vi "io_bin_data_PCfile_to_instrument.vi"(7 "Source File":path, 8 "error in":errorcluster, 10 "Command (none)":string, 11 "VISA resource name":refnum<visa-resource-name>) -> (0 "error out":errorcluster, 3 "VISA resource name out":refnum<visa-resource-name>)   [LabVIEW 2014, in "rszvl_rsidr_core.lvlib"]
uses:
  rszvl_rsidr_core.lvlib
  type_Error_Codes.ctl
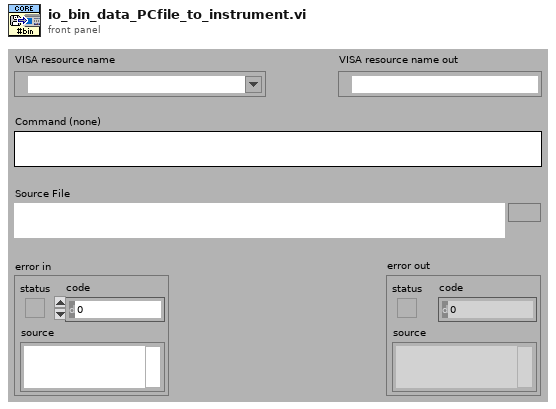
[diagram p1: front panel]
types:
  T1 = enum16{"open", "replace", "create", "open or create", "replace or create", "replace or create with confirmation"}
  T2 = typedef "rszvl_rsidr_core.lvlib/type_Error_Codes.ctl" = enum16{"No_error", "VISA_err_ResourceNotFound", "VISA_err_Timeout", "VISA_warn_MoreDataAvailable", "RS_err_MissingCallback", "RS_err_InvalidAttribute", "RS_err_InvalidValue", "RS_err_UnknownResource", "RS_err_AlreadyInitialized", "RS_err_InstrumentStatus", "RS_err_BadRepCapName", "RS_err_TypesMismatch", "RS_err_ValueNotSupported", "RS_err_InvalidRngTable", "RS_err_IDqueryFail", "RS_err_UnexpResponse", "VISA_warn_ConfigNotLoaded", "RS_err_AttributeNotReadable", "RS_err_AttributeNotWritable", "RS_err_InstrumentType", "RS_err_InstrumentOption", "VISA_err_InvalidSize", "RS_err_ReliabilityIndicator", "VISA_warn_UnknownStatus", "VISA_warn_TermCharRead", "VISA_err_IO_error"}
  T3 = typedef "rszvl_rsidr_core.lvlib/type_Session_Data.ctl" = cluster{"Instr type":string, "Instr type for err. msg.":string, "Installed Options":string[], "OPC Timeout":i32, "Query Instrument Status":bool, "Check Range":bool, "Check Options":bool, "Add LF to Write":bool, "Simulate":bool, "Logging":bool, "Logging params":variant, "Interface Type":enum16{"Unknown", "GPIB", "VXI", "GPIB_VXI", "ASRL", "PXI", "TCPIP", "USB", "SOCKET"}, "Fast Sweep":i32, "AdditionalFlags":i32, "WaitBeforeWrite":i32, "WaitBeforeRead":i32, "BinDataChunkSize":i64}
  T4 = enum16{"Unknown", "GPIB", "VXI", "GPIB_VXI", "ASRL", "PXI", "TCPIP", "USB", "SOCKET"}
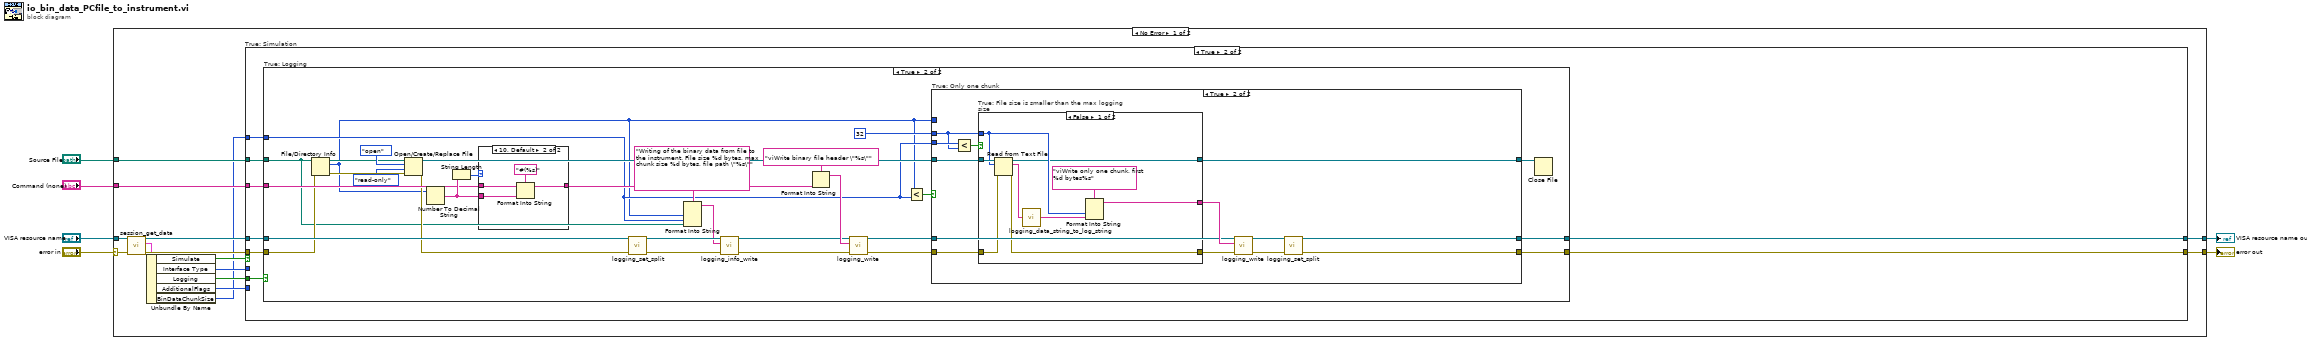
[diagram p0: block diagram]
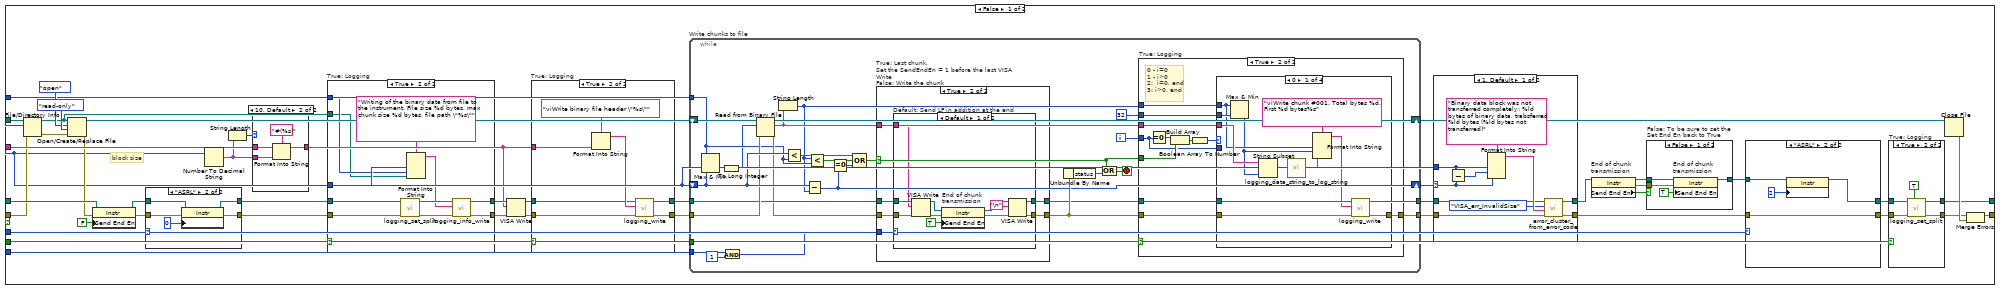
[diagram p2: hidden frame]
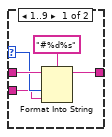
[diagram p7: hidden frame]
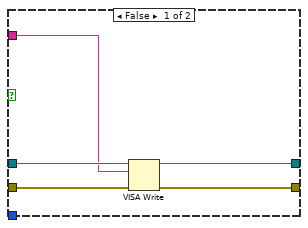
[diagram p9: hidden frame]
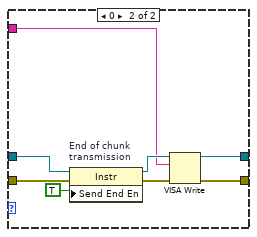
[diagram p10: hidden frame]
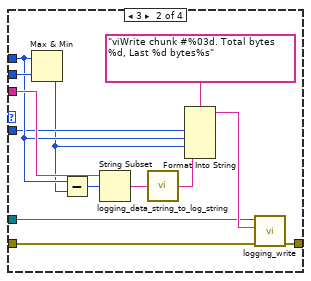
[diagram p12: hidden frame]
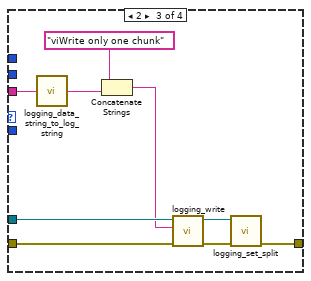
[diagram p13: hidden frame]
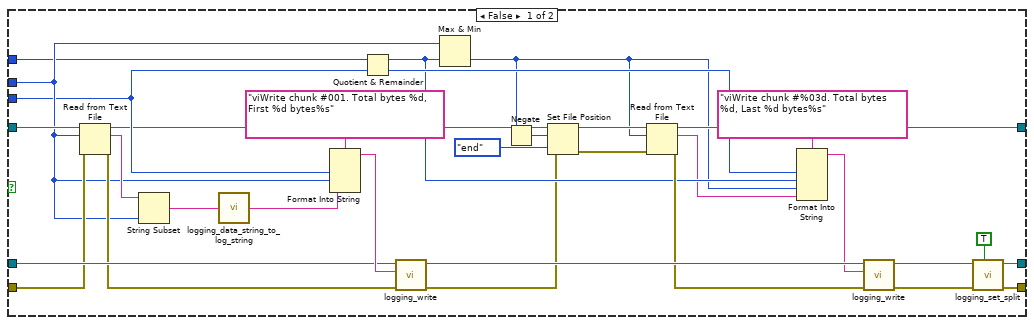
[diagram p18: hidden frame]
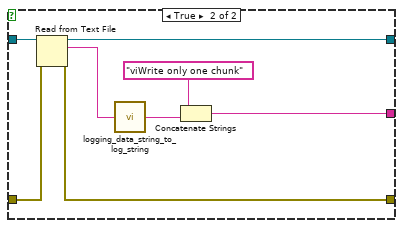
[diagram p19: hidden frame]
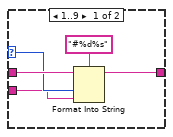
[diagram p20: hidden frame]
diagram:
  n1 = case shown="No Error" "error in" {
    selector: "error in" -> [w18 w348]
    tunnel: "Source File" -> [w20 _]
    tunnel: "Command (none)" -> [w19 _]
    tunnel: "VISA resource name" -> [w17 w349]
    tunnel: [w12 w348] -> w3
    tunnel: [w11 w349] -> w2
    frame No Error {
      n2 = call "session_get_data.vi"("error in"=w18, "VISA resource name"=w17) -> ("error out"=w16:errorcluster, "Session User Data out"=w14:T3, "VISA resource name out"=w15:refnum<visa-resource-name>)  [unwired: 7 in]
      n3 = Unbundle By Name(w14) -> ("Simulate"=w10:bool, "Interface Type"=w9:T4, "Logging"=w13:bool, "AdditionalFlags"=w8:i32, "BinDataChunkSize"=w7:i64)
      n4 = case "True: Simulation" shown="True" w10 {
        tunnel: w16 -> [w49 w241]
        tunnel: w15 -> [w65 w240]
        tunnel: w20 -> [w56 w239]
        tunnel: w19 -> [w52 w238]
        tunnel: [w29 w242] -> w11
        tunnel: [w30 w243] -> w12
        tunnel: w13 -> [w34 w244]
        tunnel: w7 -> [w35 w237]
        tunnel: w9 -> [w22 _]
        tunnel: w8 -> [w21 _]
        frame False {
          # "block size"
          n5 = File/Directory Info(path=w56, error in=w49) -> (path out=w44:path, size=w45:i64, error out=w53:errorcluster)  [unwired: 4 out]
          n6 = Open/Create/Replace File(file path (use dialog)=w44, error in=w53, operation (0:open)=T1."open", access (0:read/write)=enum16{"read/write", "read-only", "write-only"}."read-only") -> (refnum out=w62:refnum<file>, error out=w48:errorcluster)  [unwired: 2 in, 1 out]
          n7 = property on="Property Node" class="Instr"(reference=w65, error in=w48, "Send End En"=FALSE ("Message Based Settings:Send End Enable")) -> (reference out=w54:refnum<visa-resource-name>, error out=w55:errorcluster)
          n8 = case "4: ASRL" shown="\"ASRL\"" w22 {
            tunnel: w55 -> [w230 w235]
            tunnel: w54 -> [w231 w234]
            tunnel: [w231 w233] -> w47
            tunnel: [w230 w232] -> w46
            frame Default {
            }
            frame "ASRL" {
              n9 = property on="Property Node" class="Instr"(reference=w234, error in=w235, "Serial Settings:End Mode for Reads"=u16 0 ("ASRL End In")) -> (reference out=w233:refnum<visa-resource-name>, error out=w232:errorcluster)
            }
          }
          n10 = Number To Decimal String(number=w45) -> (decimal integer string=w51:string)  [unwired: 1 in]
          n11 = String Length(string=w51) -> (length=w50:i32)
          n12 = case shown="10, Default" w50 {
            selector: w50 -> [w102 _]
            tunnel: w52 -> [w103 w107]
            tunnel: w51 -> [w101 w105]
            tunnel: [w100 w106] -> w37
            frame 1..9 {
              n13 = Format Into String(format string="#%d%s", initial string=w103, w102, w101) -> (resulting string=w100:string)  [unwired: 1 in, 1 out]
            }
            frame 10, Default {
              n14 = Format Into String(format string="#(%s)", initial string=w107, w105) -> (resulting string=w106:string)  [unwired: 1 in, 1 out]
            }
          }
          n15 = case "True: Logging" shown="True" w34 {
            tunnel: w46 -> [w88 w99]
            tunnel: w47 -> [w87 w98]
            tunnel: w35 -> [_ w95]
            tunnel: [w88 w91] -> w41
            tunnel: [w87 w90] -> w42
            tunnel: w45 -> [_ w96]
            tunnel: w44 -> [_ w94]
            frame False {
            }
            frame True {
              n16 = call "logging_set_split.vi"("error in"=w99, "VISA resource name"=w98) -> ("error out"=w93:errorcluster, "VISA resource name out"=w92:refnum<visa-resource-name>)  [unwired: 8 in]
              n17 = Format Into String(format string="Writing of the binary data from file to the instrument. File size %d bytes, max chunk size %d bytes, file path \"%s\"", w96, w95, w94) -> (resulting string=w89:string)  [unwired: 2 in, 1 out]
              n18 = call "logging_info_write.vi"("error in"=w93, "String to write"=w89, "VISA resource name"=w92) -> ("error out"=w91:errorcluster, "VISA resource name out"=w90:refnum<visa-resource-name>)  [unwired: 7 in]
            }
          }
          n19 = VISA Write(VISA resource name=w42, write buffer=w37, error in (no error)=w41) -> (VISA resource name out=w39:refnum<visa-resource-name>, error out=w40:errorcluster)  [unwired: 1 out]
          n20 = case "True: Logging" shown="True" w34 {
            tunnel: w40 -> [w79 w84]
            tunnel: w39 -> [w78 w83]
            tunnel: [w79 w82] -> w38
            tunnel: [w78 w81] -> w36
            tunnel: w37 -> [_ w80]
            frame False {
            }
            frame True {
              n21 = Format Into String(format string="viWrite binary file header \"%s\"", w80) -> (resulting string=w85:string)  [unwired: 2 in, 1 out]
              n22 = call "logging_write.vi"("error in"=w84, "String to write"=w85, "VISA resource name"=w83) -> ("error out"=w82:errorcluster, "VISA resource name out"=w81:refnum<visa-resource-name>)  [unwired: 7 in]
            }
          }
          n23 = while "Write chunks to file" {
            tunnel: w38 -> [w142]
            tunnel: w36 -> [w134]
            tunnel: w35 -> [w125]
            shift-right: [w123] -> w59
            shift-left: w45 -> [w145]
            tunnel: [w140] -> w58
            shift-right: [w143] -> w61
            shift-left: w62 -> [w144]
            tunnel: w34 -> [w138]
            tunnel: [w130] -> w28
            tunnel: w21 -> [w127]
            i -> [w135]
            stop <- w146 stop-if-true
            n24 = Max & Min(x=w125, y=w145) -> (min(x,y)=w141:i64)  [unwired: 1 out]
            n25 = To Long Integer(number=w141) -> (32bit integer=w124:i32)
            n26 = And(x=w127, y=1 ("x")) -> (x .and. y?=w126:i32)
            n27 = Read from Binary File(8:w142, 10:w124, 11:w144) -> (0:w133:errorcluster, 2:w131:string, 3:w143:refnum<file>)  [unwired: 3 in, 1 out]
            n28 = String Length(string=w131) -> (length=w121:i32)
            n29 = Less?(x=w145, y=w125) -> (x < y?=w137:bool)
            n30 = Subtract(x=w145, y=w121) -> (x-y=w123:i64)
            n31 = Less?(x=w121, y=w125) -> (x < y?=w136:bool)
            n32 = Equal To 0?(x=w123) -> (x = 0?=w122:bool)
            n33 = Compound Arithmetic op=OR(w137, w136, w122) -> (w129:bool)
            n34 = case "True: Last chunk,\nSet the SendEndEn = 1 before the last VISA Write\nFalse: Write the chunk" shown="True" w129 {
              tunnel: w134 -> [w151 w158]
              tunnel: w133 -> [w152 w157]
              tunnel: [w150 w156] -> w132
              tunnel: w131 -> [w148 w155]
              tunnel: [w149 w154] -> w130
              tunnel: w126 -> [_ w153]
              frame False {
                n35 = VISA Write(VISA resource name=w151, write buffer=w148, error in (no error)=w152) -> (VISA resource name out=w149:refnum<visa-resource-name>, error out=w150:errorcluster)  [unwired: 1 out]
              }
              frame True {
                n36 = case "Default: Send LF in addition at the end" shown="Default" w153 {
                  tunnel: w158 -> [w163 w177]
                  tunnel: w157 -> [w164 w176]
                  tunnel: [w167 w173] -> w156
                  tunnel: w155 -> [w160 w172]
                  tunnel: [w166 w171] -> w154
                  frame Default {
                    n37 = VISA Write(VISA resource name=w163, write buffer=w160, error in (no error)=w164) -> (VISA resource name out=w161:refnum<visa-resource-name>, error out=w162:errorcluster)  [unwired: 1 out]
                    n38 = property on="End of chunk\ntransmission" class="Instr"(reference=w161, error in=w162, "Send End En"=TRUE ("Message Based Settings:Send End Enable")) -> (reference out=w168:refnum<visa-resource-name>, error out=w169:errorcluster)
                    n39 = VISA Write(VISA resource name=w168, write buffer="\n" ("Line Feed Constant"), error in (no error)=w169) -> (VISA resource name out=w166:refnum<visa-resource-name>, error out=w167:errorcluster)  [unwired: 1 out]
                  }
                  frame 0 {
                    n40 = property on="End of chunk\ntransmission" class="Instr"(reference=w177, error in=w176, "Send End En"=TRUE ("Message Based Settings:Send End Enable")) -> (reference out=w174:refnum<visa-resource-name>, error out=w175:errorcluster)
                    n41 = VISA Write(VISA resource name=w174, write buffer=w172, error in (no error)=w175) -> (VISA resource name out=w171:refnum<visa-resource-name>, error out=w173:errorcluster)  [unwired: 1 out]
                  }
                }
              }
            }
            n42 = Unbundle By Name(w132) -> ("status"=w147:bool)
            n43 = Compound Arithmetic op=OR(w129, w147) -> (w146:bool)
            n44 = case "True: Logging" shown="True" w138 {
              tunnel: w132 -> [w178 w189]
              tunnel: w130 -> [_ w188]
              tunnel: [w178 w187] -> w140
              tunnel: w131 -> [_ w186]
              tunnel: w121 -> [_ w185]
              tunnel: 32 ("length (rest)") -> [_ w184]
              tunnel: w129 -> [_ w183]
              tunnel: w135 -> [_ w179]
              frame False {
              }
              frame True {
                # "0 - i=0\n1 - i>0\n2:  i=0, end\n3: i>0, end"
                n45 = Equal To 0?(x=w179) -> (x = 0?=w182:bool)
                n46 = Build Array(w182, w183) -> (w181:bool[])
                n47 = Boolean Array To Number(Boolean array=w181) -> (number=w180:u32)
                n48 = case shown="0" w180 {
                  tunnel: w189 -> [w198 w211 w222 w223]
                  tunnel: w188 -> [w197 w210 w221 _]
                  tunnel: [w196 w201 w214 w223] -> w187
                  tunnel: w186 -> [w195 w209 w220 _]
                  tunnel: w185 -> [w192 w206 _ _]
                  tunnel: w184 -> [w193 w207 _ _]
                  tunnel: w179 -> [_ w204 _ _]
                  frame 0 {
                    n49 = Max & Min(x=w192, y=w193) -> (min(x,y)=w191:i32)  [unwired: 1 out]
                    n50 = String Subset(string=w195, length (rest)=w191) -> (substring=w194:string)  [unwired: 1 in]
                    n51 = call "logging_data_string_to_log_string.vi"("Raw string to log"=w194) -> ("Result log string"=w190:string)  [unwired: 4 in]
                    n52 = Format Into String(format string="viWrite chunk #001. Total bytes %d, First %d bytes%s", w192, w191, w190) -> (resulting string=w199:string)  [unwired: 2 in, 1 out]
                    n53 = call "logging_write.vi"("error in"=w198, "String to write"=w199, "VISA resource name"=w197) -> ("error out"=w196:errorcluster)  [unwired: 7 in, 1 out]
                  }
                  frame 3 {
                    n54 = Max & Min(x=w206, y=w207) -> (min(x,y)=w203:i32)  [unwired: 1 out]
                    n55 = Subtract(x=w206, y=w203) -> (x-y=w205:i32)
                    n56 = String Subset(string=w209, offset (0)=w205) -> (substring=w208:string)  [unwired: 1 in]
                    n57 = call "logging_data_string_to_log_string.vi"("Raw string to log"=w208) -> ("Result log string"=w202:string)  [unwired: 4 in]
                    n58 = Format Into String(format string="viWrite chunk #%03d. Total bytes %d, Last %d bytes%s", w204, w206, w203, w202) -> (resulting string=w212:string)  [unwired: 2 in, 1 out]
                    n59 = call "logging_write.vi"("error in"=w211, "String to write"=w212, "VISA resource name"=w210) -> ("error out"=w201:errorcluster)  [unwired: 7 in, 1 out]
                  }
                  frame 2 {
                    n60 = call "logging_data_string_to_log_string.vi"("Raw string to log"=w220) -> ("Result log string"=w217:string)  [unwired: 4 in]
                    n61 = Concatenate Strings("viWrite only one chunk" ("format string"), w217) -> (w218:string)
                    n62 = call "logging_write.vi"("error in"=w222, "String to write"=w218, "VISA resource name"=w221) -> ("error out"=w216:errorcluster, "VISA resource name out"=w215:refnum<visa-resource-name>)  [unwired: 7 in]
                    n63 = call "logging_set_split.vi"("error in"=w216, "VISA resource name"=w215) -> ("error out"=w214:errorcluster)  [unwired: 8 in, 1 out]
                  }
                  frame Default {
                  }
                }
              }
            }
          }
          n64 = case shown="1, Default" w59 {
            selector: w59 -> [w113 _]
            tunnel: w58 -> [w116 w120]
            tunnel: [w117 w120] -> w43
            tunnel: w45 -> [w115 _]
            tunnel: w28 -> [w111 w119]
            tunnel: [w110 w119] -> w27
            frame 1, Default {
              n65 = Subtract(x=w115, y=w113) -> (x-y=w114:i64)
              n66 = Format Into String(format string="Binary data block was not transferred completely: %ld bytes of binary data, trabsferred %ld bytes (%ld bytes not transferred)" ("error message (\"\")"), w115, w114, w113) -> (resulting string=w112:string)  [unwired: 2 in, 1 out]
              n67 = call "error_cluster_from_error_code.vi"("error in"=w116, "error message (\"\")"=w112, "Error Enum in"=type_Error_Codes."VISA_err_InvalidSize", "VISA resource name"=w111) -> ("error out"=w117:errorcluster, "VISA resource name out"=w110:refnum<visa-resource-name>)  [unwired: 6 in]
            }
            frame 0 {
            }
          }
          n68 = property on="End of chunk\ntransmission" class="Instr"(reference=w27) -> (reference out=w26:refnum<visa-resource-name>, error out=w24:errorcluster, "Send End En"=w25:bool)  [unwired: 1 in]
          n69 = case "False: To be sure to set the\nSet End En back to True" shown="False" w25 {
            tunnel: w26 -> [w69 w70]
            tunnel: w24 -> [w68 _]
            tunnel: [w67 w70] -> w23
            frame False {
              n70 = property on="End of chunk\ntransmission" class="Instr"(reference=w69, error in=w68, "Send End En"=TRUE ("Message Based Settings:Send End Enable")) -> (reference out=w67:refnum<visa-resource-name>)  [unwired: 1 out]
            }
            frame True {
            }
          }
          n71 = case "4: ASRL" shown="\"ASRL\"" w22 {
            tunnel: w23 -> [w224 w228]
            tunnel: [w224 w226] -> w32
            tunnel: w43 -> [w225 w227]
            tunnel: [w225 w227] -> w33
            frame Default {
            }
            frame "ASRL" {
              n72 = property on="Property Node" class="Instr"(reference=w228, "Serial Settings:End Mode for Reads"=u16 2 ("ASRL End In")) -> (reference out=w226:refnum<visa-resource-name>)  [unwired: 1 in, 1 out]
            }
          }
          n73 = case "True: Logging" shown="True" w34 {
            tunnel: w33 -> [w72 w77]
            tunnel: w32 -> [w71 w76]
            tunnel: [w72 w75] -> w31
            tunnel: [w71 w74] -> w29
            frame False {
            }
            frame True {
              n74 = call "logging_set_split.vi"("Evaluate section error (F)"=TRUE, "error in"=w77, "VISA resource name"=w76) -> ("error out"=w75:errorcluster, "VISA resource name out"=w74:refnum<visa-resource-name>)  [unwired: 7 in]
            }
          }
          n75 = Close File(refnum=w61) -> (error out=w60:errorcluster)  [unwired: 1 in, 1 out]
          n76 = Merge Errors(w31, w60) -> (w30:errorcluster)
        }
        frame True {
          n77 = case "True: Logging" shown="True" w244 {
            tunnel: w241 -> [w246 w266]
            tunnel: w240 -> [w245 w268]
            tunnel: [w246 w248] -> w243
            tunnel: [w245 w247] -> w242
            tunnel: w239 -> [_ w264]
            tunnel: w238 -> [_ w271]
            tunnel: w237 -> [_ w254]
            frame False {
            }
            frame True {
              n78 = File/Directory Info(path=w264, error in=w266) -> (path out=w274:path, size=w251:i64, error out=w275:errorcluster)  [unwired: 4 out]
              n79 = Open/Create/Replace File(file path (use dialog)=w274, error in=w275, operation (0:open)=T1."open", access (0:read/write)=enum16{"read/write", "read-only", "write-only"}."read-only") -> (refnum out=w255:refnum<file>, error out=w265:errorcluster)  [unwired: 2 in, 1 out]
              n80 = Number To Decimal String(number=w251) -> (decimal integer string=w273:string)  [unwired: 1 in]
              n81 = String Length(string=w273) -> (length=w272:i32)
              n82 = case shown="10, Default" w272 {
                selector: w272 -> [w341 _]
                tunnel: w271 -> [w342 w346]
                tunnel: w273 -> [w340 w344]
                tunnel: [w339 w345] -> w258
                frame 1..9 {
                  n83 = Format Into String(format string="#%d%s", initial string=w342, w341, w340) -> (resulting string=w339:string)  [unwired: 1 in, 1 out]
                }
                frame 10, Default {
                  n84 = Format Into String(format string="#(%s)", initial string=w346, w344) -> (resulting string=w345:string)  [unwired: 1 in, 1 out]
                }
              }
              n85 = call "logging_set_split.vi"("error in"=w265, "VISA resource name"=w268) -> ("error out"=w269:errorcluster, "VISA resource name out"=w270:refnum<visa-resource-name>)  [unwired: 8 in]
              n86 = Format Into String(format string="Writing of the binary data from file to the instrument. File size %d bytes, max chunk size %d bytes, file path \"%s\"", w251, w254, w264) -> (resulting string=w263:string)  [unwired: 2 in, 1 out]
              n87 = call "logging_info_write.vi"("error in"=w269, "String to write"=w263, "VISA resource name"=w270) -> ("error out"=w260:errorcluster, "VISA resource name out"=w259:refnum<visa-resource-name>)  [unwired: 7 in]
              n88 = Format Into String(format string="viWrite binary file header \"%s\"", w258) -> (resulting string=w261:string)  [unwired: 2 in, 1 out]
              n89 = call "logging_write.vi"("error in"=w260, "String to write"=w261, "VISA resource name"=w259) -> ("error out"=w253:errorcluster, "VISA resource name out"=w252:refnum<visa-resource-name>)  [unwired: 7 in]
              n90 = Less?(x=w251, y=w254) -> (x < y?=w257:bool)
              n91 = case "True: Only one chunk" shown="True" w257 {
                tunnel: 32 ("length (rest)") -> [w297 w314]
                tunnel: w255 -> [w303 w321]
                tunnel: w253 -> [w302 w317]
                tunnel: w254 -> [w295 w320]
                tunnel: w252 -> [w304 w315]
                tunnel: [w279 w310] -> w248
                tunnel: [w278 w309] -> w247
                tunnel: w251 -> [w296 _]
                tunnel: [w294 w313] -> w249
                frame False {
                  n92 = Read from Text File(file (use dialog)=w303, count=w297, error in=w302) -> (refnum out=w289:refnum<file>, text=w300:string, error out=w301:errorcluster)  [unwired: 1 in, 1 out]
                  n93 = String Subset(string=w300, length (rest)=w297) -> (substring=w307:string)  [unwired: 1 in]
                  n94 = call "logging_data_string_to_log_string.vi"("Raw string to log"=w307) -> ("Result log string"=w308:string)  [unwired: 4 in]
                  n95 = Format Into String(format string="viWrite chunk #001. Total bytes %d, First %d bytes%s", w295, w297, w308) -> (resulting string=w306:string)  [unwired: 2 in, 1 out]
                  n96 = Quotient & Remainder(x=w296, y=w295) -> (x-y*floor(x/y)=w290:i64, floor(x/y)=w291:i64)
                  n97 = call "logging_write.vi"("error in"=w301, "String to write"=w306, "VISA resource name"=w304) -> ("error out"=w288:errorcluster, "VISA resource name out"=w299:refnum<visa-resource-name>)  [unwired: 7 in]
                  n98 = Max & Min(x=w297, y=w290) -> (min(x,y)=w283:i64)  [unwired: 1 out]
                  n99 = Negate(x=w283) -> (-x=w285:i64)
                  n100 = Set File Position(offset (in bytes) (0)=w285, refnum=w289, from (0:start)=enum16{"start", "end", "current"}."end", error in=w288) -> (refnum out=w284:refnum<file>, error out=w287:errorcluster)
                  n101 = Read from Text File(file (use dialog)=w284, count=w283, error in=w287) -> (refnum out=w294:refnum<file>, text=w282:string, error out=w293:errorcluster)  [unwired: 1 in, 1 out]
                  n102 = Format Into String(format string="viWrite chunk #%03d. Total bytes %d, Last %d bytes%s", w291, w290, w283, w282) -> (resulting string=w292:string)  [unwired: 2 in, 1 out]
                  n103 = call "logging_write.vi"("error in"=w293, "String to write"=w292, "VISA resource name"=w299) -> ("error out"=w281:errorcluster, "VISA resource name out"=w280:refnum<visa-resource-name>)  [unwired: 7 in]
                  n104 = call "logging_set_split.vi"("Evaluate section error (F)"=TRUE, "error in"=w281, "VISA resource name"=w280) -> ("error out"=w279:errorcluster, "VISA resource name out"=w278:refnum<visa-resource-name>)  [unwired: 7 in]
                }
                frame True {
                  n105 = Less?(x=w320, y=w314) -> (x < y?=w319:bool)
                  n106 = case "True: File size is smaller than the max logging size" shown="False" w319 {
                    tunnel: w321 -> [w330 w336]
                    tunnel: [w327 w334] -> w318
                    tunnel: w317 -> [w329 w333]
                    tunnel: [w323 w332] -> w316
                    tunnel: w314 -> [w326 _]
                    tunnel: [w322 w331] -> w313
                    frame False {
                      n107 = Read from Text File(file (use dialog)=w330, count=w326, error in=w329) -> (refnum out=w322:refnum<file>, text=w325:string, error out=w323:errorcluster)  [unwired: 1 in, 1 out]
                      n108 = call "logging_data_string_to_log_string.vi"("Raw string to log"=w325) -> ("Result log string"=w324:string)  [unwired: 4 in]
                      n109 = Format Into String(format string="viWrite only one chunk, first %d bytes%s", w326, w324) -> (resulting string=w327:string)  [unwired: 2 in, 1 out]
                    }
                    frame True {
                      n110 = Read from Text File(file (use dialog)=w336, error in=w333) -> (refnum out=w331:refnum<file>, text=w335:string, error out=w332:errorcluster)  [unwired: 2 in, 1 out]
                      n111 = call "logging_data_string_to_log_string.vi"("Raw string to log"=w335) -> ("Result log string"=w337:string)  [unwired: 4 in]
                      n112 = Concatenate Strings("viWrite only one chunk" ("format string"), w337) -> (w334:string)
                    }
                  }
                  n113 = call "logging_write.vi"("error in"=w316, "String to write"=w318, "VISA resource name"=w315) -> ("error out"=w312:errorcluster, "VISA resource name out"=w311:refnum<visa-resource-name>)  [unwired: 7 in]
                  n114 = call "logging_set_split.vi"("error in"=w312, "VISA resource name"=w311) -> ("error out"=w310:errorcluster, "VISA resource name out"=w309:refnum<visa-resource-name>)  [unwired: 8 in]
                }
              }
              n115 = Close File(refnum=w249) -> ()  [unwired: 1 in, 2 out]
            }
          }
        }
      }
    }
    frame Error {
    }
  }
  "error out" <- w3
  "VISA resource name out" <- w2
